vi "Teleop.vi"(10 "Match Info":T1={"Autonomous Elapsed Seconds"=0.0, "TeleOp Elapsed Seconds"=0.0, "Disabled Elapsed Seconds"=0.0, "Visited Autonomous"=FALSE, "Visited TeleOp"=FALSE, "Visited Disabled"=FALSE, "Autonomous Settings"={"Autonomous Style"=enum."Independent", "VI Refnum"=refnum}}, 11 "Call Context":T2) -> ()   [LabVIEW 2014]
doc: "This VI is called for each TeleOp packet received from the DS where the robot is not disabled. It is often used to read from the joysticks and update I/O or to update setpoints for timed control loops. It should complete and return within 20 milliseconds or it may miss DS packets."
uses:
  <vilib>/Rock Robotics/WPI/DriverStation/WPI_DriverStationDerivedRobotMode.ctl
  <vilib>/Rock Robotics/WPI/DriverStation/WPI_DriverStationMatch Info.ctl
  <vilib>/Rock Robotics/Network Tables/SD Read Boolean.vi
  <vilib>/Rock Robotics/Network Tables/SD Read Number.vi
  <vilib>/Rock Robotics/WPI/Joystick/WPI_JoystickGetSetRefNum.vi
  <vilib>/Rock Robotics/Network Tables/SD Write Boolean Array.vi
  <vilib>/Rock Robotics/Network Tables/SD Write Numeric Array.vi
  <vilib>/Rock Robotics/Network Tables/SD Write Boolean.vi
  Robot Global Data.vi
  <vilib>/Rock Robotics/WPI/RobotDrive/WPI_RobotDriveGetSetRefNum.vi
panel:
  out "Angle":dbl
  out "Sample Slider 0":dbl(slide) scale=0.0..5.0
  out "Sample Boolean 1":bool
  out "Sample Boolean 0":bool
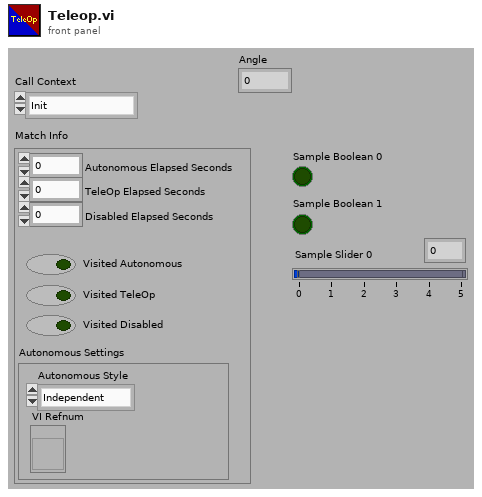
[diagram p1: front panel]
types:
  T1 = typedef "WPI_DriverStationMatch Info.ctl" = cluster{"Autonomous Elapsed Seconds":dbl, "TeleOp Elapsed Seconds":dbl, "Disabled Elapsed Seconds":dbl, "Visited Autonomous":bool, "Visited TeleOp":bool, "Visited Disabled":bool, "Autonomous Settings":cluster{"Autonomous Style":enum16{"Iterative", "Independent"}, "VI Refnum":refnum<vi>}}
  T2 = typedef "WPI_DriverStationDerivedRobotMode.ctl" = enum16{"Init", "Execute", "Stop"}
  T3 = typedef "WPI_RobotDriveDevRef.ctl" = cluster{"DevStatus":errorcluster, "Motors[]":T4[], "Square Inputs":bool, "Max Output":dbl}
  T4 = typedef "WPI_MotorControlDeviceRef.ctl" = cluster{"DeviceStatus":errorcluster, "Type":T5, "PWM":cluster{"Controller":T6, "PWM Channel":T7, "DeadBand":T8}, "CAN":cluster{"Device Number":u8, "Control Mode":T9, "Semaphore":T10, "Max Vout":dbl, "TalonSRX Control Mode":T11}, "Invert":bool, "TransformRef":T12, "InvTransformRef":T12}
  T5 = typedef "WPI_MotorControlType.ctl" = enum16{"PWM", "CAN", "CANTalonSRX"}
  T6 = typedef "FPGA_TypedefDigitalModule.ctl" = enum16{"Controller 1"}
  T7 = typedef "FPGA_DIOPWMChannel.ctl" = enum8{"PWM 0", "PWM 1", "PWM 2", "PWM 3", "PWM 4", "PWM 5", "PWM 6", "PWM 7", "PWM 8", "PWM 9", "PWM MXP 0", "PWM MXP 1", "PWM MXP 2", "PWM MXP 3", "PWM MXP 4", "PWM MXP 5", "PWM MXP 6", "PWM MXP 7", "PWM MXP 8", "PWM MXP 9", "Invalid"}
  T8 = typedef "WPI_PWMDeadband.ctl" = cluster{"Name":string, "maxPositivePwm":i32, "minPositivePwm":i32, "centerPwm":i32, "maxNegativePwm":i32, "minNegativePwm":i32, "angularRange":u16}
  T9 = typedef "WPI_CANJaguar_ControlMode.ctl" = enum8{"Percent VBus", "Current", "Speed", "Position", "Voltage"}
  T10 = typedef "Semaphore RefNum" = refnum<k1>
  T11 = typedef "WPI_CANTalonSRX_APIControlMode.ctl" = enum8{"Percent VBus", "Speed", "Position", "Slave", "Unchanged / Invalid"}
  T12 = typedef "WPI_PWMTransform_ConPane.ctl" = refnum<vi>
  T13 = typedef "WPI_JoystickDevRef.ctl" = cluster{"Device":T14}
  T14 = typedef "WPI_JoystickDeviceEnum.ctl" = enum16{"USB 0", "USB 1", "USB 2", "USB 3", "USB 4", "USB 5"}
  T15 = typedef "WPI_DigitalInputDevRef.ctl" = cluster{"DevStatus":errorcluster, "DIO Channel":T16, "Controller":T6}
  T16 = typedef "FPGA_DIOChannel.ctl" = enum8{"DIO 0", "DIO 1", "DIO 2", "DIO 3", "DIO 4", "DIO 5", "DIO 6", "DIO 7", "DIO 8", "DIO 9", "DIO MXP 0", "DIO MXP 1", "DIO MXP 2", "DIO MXP 3", "DIO MXP 4", "DIO MXP 5", "DIO MXP 6", "DIO MXP 7", "DIO MXP 8", "DIO MXP 9", "DIO MXP 10", "DIO MXP 11", "DIO MXP 12", "DIO MXP 13", "DIO MXP 14", "DIO MXP 15", "Invalid"}
  T17 = typedef "WPI_GyroDevRef.ctl" = cluster{"DevStatus":errorcluster, "Analog Module":T18, "Analog Channel":T19, "Offset":dbl, "Gain (VoltsPerDegree/Second)":dbl}
  T18 = typedef "FPGA_TypedefAnalogModule.ctl" = enum16{"Controller 1"}
  T19 = typedef "FPGA_AIChannel.ctl" = enum8{"AI 0", "AI 1", "AI 2", "AI 3", "AI MXP 0", "AI MXP 1", "AI MXP 2", "AI MXP 3", "Invalid"}
  T20 = typedef "WPI_EncoderDevRef.ctl" = cluster{"DevStatus":errorcluster, "EncoderIndex":T21, "CounterIndex":T22, "DistancePerCount":dbl, "Decoding Type":T23}
  T21 = typedef "FPGA_EncoderIdx.ctl" = enum8{"Enc 0", "Enc 1", "Enc 2", "Enc 3", "Enc 4", "Enc 5", "Enc 6", "Enc 7", "Invalid"}
  T22 = typedef "FPGA_CounterCtrSystemIndex.ctl" = enum8{"Ctr 0", "Ctr 1", "Ctr 2", "Ctr 3", "Ctr 4", "Ctr 5", "Ctr 6", "Ctr 7", "Invalid"}
  T23 = typedef "WPI_EncoderType.ctl" = enum16{"1x", "2x", "4x"}
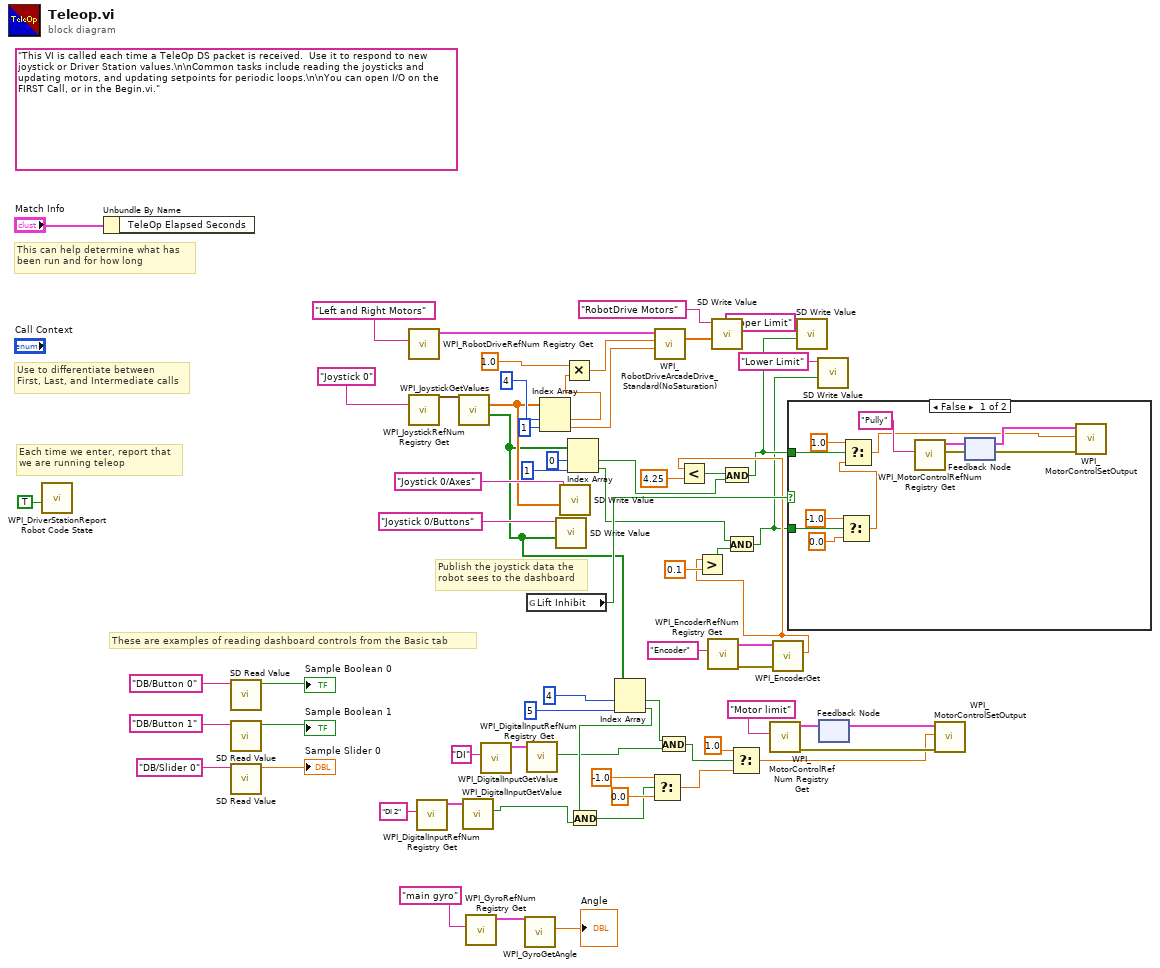
[diagram p0: block diagram]
diagram:
  (unwired) "This VI is called each time a TeleOp DS packet is received.  Use it to respond to new joystick or Driver Station values.\n\nCommon tasks include reading the joysticks and updating motors, and updating setpoints for periodic loops.\n\nYou can open I/O on the FIRST Call, or in the Begin.vi."
  # "Publish the joystick data the\nrobot sees to the dashboard"
  # "These are examples of reading dashboard controls from the Basic tab"
  # "Each time we enter, report that\nwe are running teleop"
  # "Use to differentiate between\nFirst, Last, and Intermediate calls"
  # "This can help determine what has\nbeen run and for how long"
  n1 = call <vilib>:"WPI_DriverStationReport Robot Code State.vi"("TeleOp"=TRUE ("Autonomous")) -> ()  [unwired: 10 in, 1 out]
  n2 = Unbundle By Name("Match Info") -> ()  [unwired: 1 out]
  n3 = call-poly <vilib>:"SD Read Value.vi"("Name"="DB/Button 0" ("refnum name")) -> ("Boolean"=→"Sample Boolean 0":bool)  [unwired: 8 in, 2 out]
  n4 = call-poly <vilib>:"SD Read Value.vi"("Name"="DB/Button 1" ("refnum name")) -> ("Boolean"=→"Sample Boolean 1":bool)  [unwired: 8 in, 2 out]
  n5 = call-poly <vilib>:"SD Read Value.vi"("Name"="DB/Slider 0" ("refnum name")) -> ("Numeric"=→"Sample Slider 0":dbl)  [unwired: 8 in, 2 out]
  n6 = call <vilib>:"WPI_RobotDriveRefNum Registry Get.vi"("refnum name"="Left and Right Motors") -> ("RobotDriveDevRef"=w16:T3)  [unwired: 1 in, 9 out]
  n7 = call <vilib>:"WPI_JoystickRefNum Registry Get.vi"("refnum name"="Joystick 0") -> ("JoystickDevRef"=w52:T13)  [unwired: 1 in, 9 out]
  n8 = call <vilib>:"WPI_DigitalInputRefNum Registry Get.vi"("refnum name"="DI 2") -> ("DigitalInputDevRef"=w27:T15)  [unwired: 9 in, 1 out]
  n9 = call <vilib>:"WPI_JoystickGetValues.vi"("JoystickDevRef"=w52) -> ("Buttons"=w17:bool[], "Axes"=w41:dbl[])  [unwired: 6 in, 3 out]
  n10 = call <vilib>:"WPI_DigitalInputGetValue.vi"("DigitalInputDevRef"=w27) -> ("Value"=w20:bool)  [unwired: 8 in, 2 out]
  n11 = call <vilib>:"WPI_GyroRefNum Registry Get.vi"("refnum name"="main gyro") -> ("GyroDevRef"=w56:T17)  [unwired: 9 in, 1 out]
  n12 = call <vilib>:"WPI_DigitalInputRefNum Registry Get.vi"("refnum name"="DI") -> ("DigitalInputDevRef"=w29:T15)  [unwired: 9 in, 1 out]
  n13 = call <vilib>:"WPI_GyroGetAngle.vi"("GyroDevRef"=w56) -> ("Angle"=→"Angle":dbl)  [unwired: 7 in, 3 out]
  n14 = global read "Robot Global Data.vi" "Lift Inhibit"() -> (w44:bool)
  n15 = call <vilib>:"WPI_DigitalInputGetValue.vi"("DigitalInputDevRef"=w29) -> ("Value"=w21:bool)  [unwired: 8 in, 2 out]
  n16 = Index Array(array=w41, index #1=4 ("index"), index #2=1 ("index")) -> (element #1=w19:dbl, element #2=w50:dbl)
  n17 = call-poly <vilib>:"SD Write Value.vi"("Boolean Array"=w17, "Name"="Joystick 0/Buttons") -> ()  [unwired: 8 in, 2 out]
  n18 = call-poly <vilib>:"SD Write Value.vi"("Numeric Array"=w41, "Name"="Joystick 0/Axes") -> ()  [unwired: 8 in, 2 out]
  n19 = Multiply(x=1.0 ("f"), y=w19) -> (x*y=w18:dbl)
  n20 = Index Array(array=w17, index #1=0 ("index"), index #2=1 ("index")) -> (element #1=w5:bool, element #2=w10:bool)
  n21 = Index Array(array=w17, index #1=4 ("index"), index #2=5 ("index")) -> (element #1=w25:bool, element #2=w23:bool)
  n22 = And(x=w23, y=w20) -> (x .and. y?=w22:bool)
  n23 = Select(t=-1.0, s=w22, f=0.0) -> (s? t:f=w38:dbl)
  n24 = call <vilib>:"WPI_RobotDriveArcadeDrive_Standard(NoSaturation).vi"("Y axis value"=w50, "X axis value"=w18, "RobotDriveDevRef"=w16) -> ("Motor Values"=w49:dbl[])  [unwired: 1 in, 7 out]
  n25 = And(x=w25, y=w21) -> (x .and. y?=w24:bool)
  n26 = call <vilib>:"WPI_EncoderRefNum Registry Get.vi"("refnum name"="Encoder") -> ("error out"=w14:errorcluster, "EncoderDevRef"=w13:T20)  [unwired: 9 in]
  n27 = call-poly <vilib>:"SD Write Value.vi"("Numeric Array"=w49, "Name"="RobotDrive Motors") -> ()  [unwired: 8 in, 2 out]
  n28 = Select(t=1.0, s=w24, f=w38) -> (s? t:f=w30:dbl)
  n29 = call <vilib>:"WPI_EncoderGet.vi"("error in (no error)"=w14, "EncoderDevRef"=w13) -> ("Distance"=w8:dbl)  [unwired: 4 in, 5 out]
  n30 = Less?(x=w8, y=4.25) -> (x < y?=w6:bool)
  n31 = Greater?(x=w8, y=0.1) -> (0:w9:bool)
  n32 = And(x=w6, y=w5) -> (x .and. y?=w4:bool)
  n33 = And(x=w10, y=w9) -> (x .and. y?=w3:bool)
  n34 = case shown="False" w44 {
    tunnel: w4 -> [w76 _]
    tunnel: w3 -> [w74 _]
    frame False {
      n35 = Select(t=-1.0, s=w74, f=0.0) -> (s? t:f=w72:dbl)
      n36 = Select(t=1.0, s=w76, f=w72) -> (s? t:f=w66:dbl)
      n37 = feedback #1() -> (w68:T4)  [unwired: 1 in]
      n38 = call <vilib>:"WPI_MotorControlSetOutput.vi"("Output"=w66, "MotorControlDevRef"=w68) -> ("error out"=w71:errorcluster)  [unwired: 7 in, 2 out]
      n39 = call <vilib>:"WPI_MotorControlRefNum Registry Get.vi"("error in (no error)"=w71, "refnum name"="Pully") -> ("MotorControlDevRef"=w69:T4)  [unwired: 8 in, 1 out]
      n40 = feedback-in #1(w69) -> ()
    }
    frame True {
    }
  }
  n41 = call-poly <vilib>:"SD Write Value.vi"("Boolean"=w4, "Name"="Upper Limit") -> ()  [unwired: 8 in, 2 out]
  n42 = call-poly <vilib>:"SD Write Value.vi"("Boolean"=w3, "Name"="Lower Limit") -> ()  [unwired: 8 in, 2 out]
  n43 = feedback #2() -> (w31:T4)  [unwired: 1 in]
  n44 = call <vilib>:"WPI_MotorControlSetOutput.vi"("Output"=w30, "MotorControlDevRef"=w31) -> ("error out"=w34:errorcluster)  [unwired: 7 in, 2 out]
  n45 = call <vilib>:"WPI_MotorControlRefNum Registry Get.vi"("error in (no error)"=w34, "refnum name"="Motor limit") -> ("MotorControlDevRef"=w32:T4)  [unwired: 8 in, 1 out]
  n46 = feedback-in #2(w32) -> ()
